vi "Autonomous Independent.vi"() -> ()   [LabVIEW 2015]
doc: "This VI is called when autonomous begins, and will automatically be terminated when autonomous ends. You can carry out timed or sensor driven robot movement independently without needing to return to the caller."
uses:
  <vilib>/Rock Robotics/WPI/Utilities/WPI_GetSetVariantRefNum.vi
  <vilib>/Rock Robotics/Network Tables/NT Read String.vi
  <vilib>/Rock Robotics/Network Tables/NT Write Numeric Array.vi
  <vilib>/Rock Robotics/Network Tables/NT Read Number.vi
  <vilib>/Rock Robotics/Network Tables/NT Write Number.vi
  <vilib>/addons/control/pid/pid.llb/PID (DBL).vi
  Robot Global Data.vi
  <vilib>/addons/control/pid/NI_PID_pid.lvlib
  navX Library v2/navX Library v2.lvlib
panel:
  out "E2 Rate 3":dbl
  out "E1 Rate 3":dbl
  out "Yaw 5":dbl(graph)
  out "Roll Display 3":dbl
  out "Pitch Display 3":dbl
  out "Yaw Display 3":dbl
  in  "Yaw 4":T1={"proportional gain (Kc)"=0.2, "integral time (Ti, min)"=0.0, "derivative time (Td, min)"=0.0} {"derivative time (Td, min)" format="%.3f"; "integral time (Ti, min)" format="%.3f"; "proportional gain (Kc)" format="%.3f"}
  out "Right Motor Speed  3":dbl(graph)
  out "Left Motor Speed 3":dbl(graph)
  in  "Speed Gains  3":T1={"proportional gain (Kc)"=0.65, "integral time (Ti, min)"=0.001, "derivative time (Td, min)"=0.001} {"derivative time (Td, min)" format="%.3f"; "integral time (Ti, min)" format="%.3f"; "proportional gain (Kc)" format="%.3f"}
  out "E2 Rate 2":dbl
  out "E1 Rate 2":dbl
  out "Yaw 3":dbl(graph)
  out "Roll Display 2":dbl
  out "Pitch Display 2":dbl
  out "Yaw Display 2":dbl
  in  "Yaw 2":T1={"proportional gain (Kc)"=0.2, "integral time (Ti, min)"=0.0, "derivative time (Td, min)"=0.0} {"derivative time (Td, min)" format="%.3f"; "integral time (Ti, min)" format="%.3f"; "proportional gain (Kc)" format="%.3f"}
  out "Right Motor Speed  2":dbl(graph)
  out "Left Motor Speed 2":dbl(graph)
  in  "Distance 2":dbl=120.0
  in  "Speed Gains  2":T1={"proportional gain (Kc)"=0.65, "integral time (Ti, min)"=0.001, "derivative time (Td, min)"=0.001} {"derivative time (Td, min)" format="%.3f"; "integral time (Ti, min)" format="%.3f"; "proportional gain (Kc)" format="%.3f"}
  out "Yaw Display":dbl
  out "Pitch Display":dbl
  out "Roll Display":dbl
  in  "Aiming Gains":T1={"proportional gain (Kc)"=1.0, "integral time (Ti, min)"=0.01, "derivative time (Td, min)"=0.0} {"derivative time (Td, min)" format="%.3f"; "integral time (Ti, min)" format="%.3f"; "proportional gain (Kc)" format="%.3f"}
  out "Yaw":dbl(graph)
  in  "Target Angle":dbl=30.0
  out "E1 Rate":dbl
  out "E2 Rate":dbl
  in  "Single Turn Gains":T1={"proportional gain (Kc)"=0.12, "integral time (Ti, min)"=0.0, "derivative time (Td, min)"=0.0} {"derivative time (Td, min)" format="%.3f"; "integral time (Ti, min)" format="%.3f"; "proportional gain (Kc)" format="%.3f"}
  in  "Yaw":T1={"proportional gain (Kc)"=0.2, "integral time (Ti, min)"=0.0, "derivative time (Td, min)"=0.0} {"derivative time (Td, min)" format="%.3f"; "integral time (Ti, min)" format="%.3f"; "proportional gain (Kc)" format="%.3f"}
  out "Right Motor Speed":dbl(graph)
  out "Left Motor Speed":dbl(graph)
  out "Right Motor":dbl(graph)
  out "Left Motor":dbl(graph)
  in  "Distance":dbl=120.0
  in  "Speed Gains":T1={"proportional gain (Kc)"=0.65, "integral time (Ti, min)"=0.001, "derivative time (Td, min)"=0.001} {"derivative time (Td, min)" format="%.3f"; "integral time (Ti, min)" format="%.3f"; "proportional gain (Kc)" format="%.3f"}
  out "E2 Dist":dbl
  out "E1 Dist":dbl
  # "Be sure to right-click and choose Data Operations>>Make Current Value default if you want to save the array values with the VI"
  # "Encoder Distance Traveled"
  # "Speed we are assigning the motors and Encoder Rate"
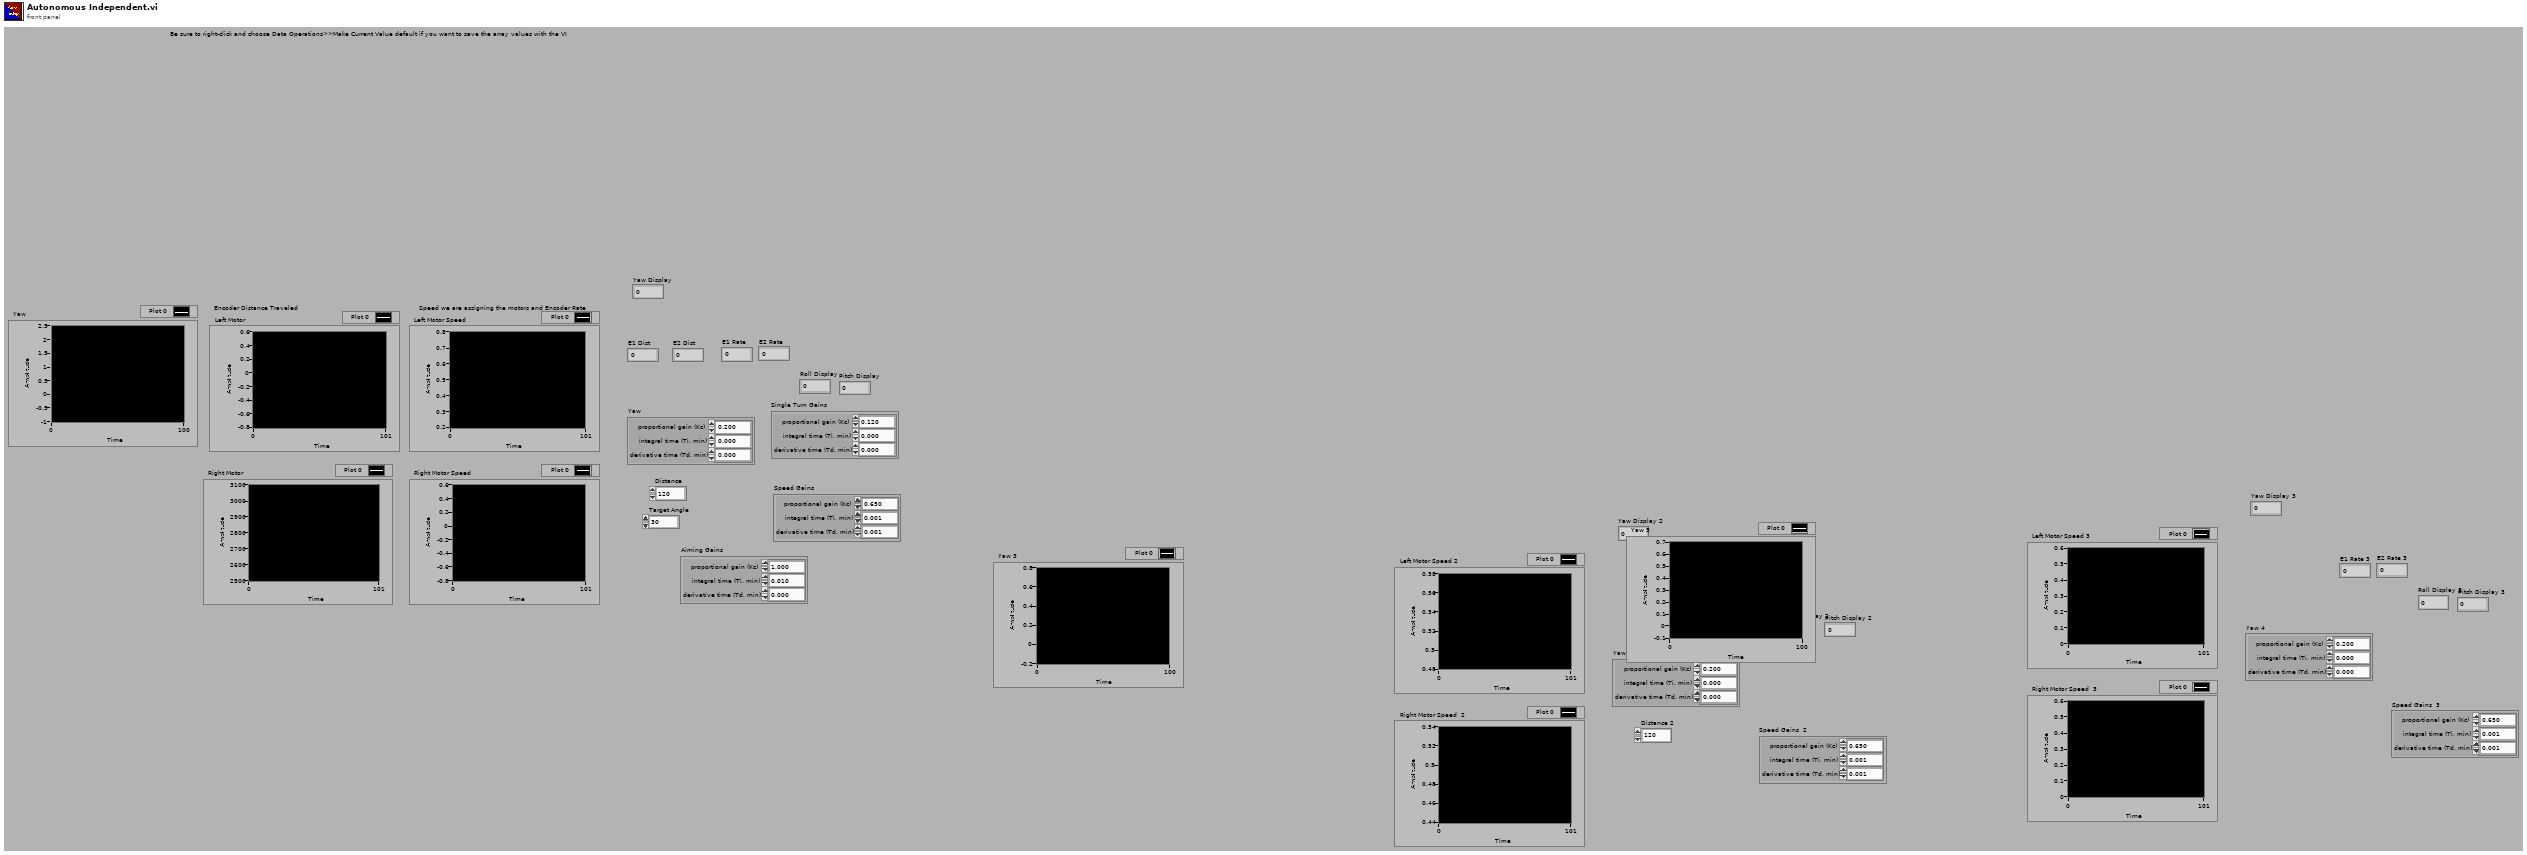
[diagram p1: front panel]
types:
  T1 = cluster{"proportional gain (Kc)":dbl, "integral time (Ti, min)":dbl, "derivative time (Td, min)":dbl}
  T2 = typedef "WPI_JoystickDevRef.ctl" = cluster{"Device":T3}
  T3 = typedef "WPI_JoystickDeviceEnum.ctl" = enum16{"USB 0", "USB 1", "USB 2", "USB 3", "USB 4", "USB 5"}
  T4 = typedef "navX Library v2.lvlib/Z900_navX_DeviceTypeDef.ctl" = cluster{"Interface":cluster{"Protocol":T5, "Update Rate (4Hz-60Hz)":u8, "navX Open TypeDef":variant}, "Notify Packet":refnum<notifier>, "Loop VI Refnum":refnum<vi>, "Ready to Close Occurrence Refnum":refnum<k4>}
  T5 = typedef "navX Library v2.lvlib/Z900_navX_ProtocolTypeDef.ctl" = enum16{"SERIAL", "I2C", "SPI"}
  T6 = typedef "WPI_EncoderDevRef.ctl" = cluster{"DevStatus":errorcluster, "EncoderIndex":T7, "CounterIndex":T8, "DistancePerCount":dbl, "Decoding Type":T9}
  T7 = typedef "FPGA_EncoderIdx.ctl" = enum8{"Enc 0", "Enc 1", "Enc 2", "Enc 3", "Enc 4", "Enc 5", "Enc 6", "Enc 7", "Invalid"}
  T8 = typedef "FPGA_CounterCtrSystemIndex.ctl" = enum8{"Ctr 0", "Ctr 1", "Ctr 2", "Ctr 3", "Ctr 4", "Ctr 5", "Ctr 6", "Ctr 7", "Invalid"}
  T9 = typedef "WPI_EncoderType.ctl" = enum16{"1x", "2x", "4x"}
  T10 = cluster{"Yaw":dbl, "Roll":dbl, "Pitch":dbl, "Heading":dbl, "Fused Heading":dbl}
  T11 = typedef "WPI_RobotDriveDevRef.ctl" = cluster{"DevStatus":errorcluster, "Motors[]":T12[], "Square Inputs":bool, "Max Output":dbl}
  T12 = typedef "WPI_MotorControlDeviceRef.ctl" = cluster{"DeviceStatus":errorcluster, "Type":T13, "PWM":cluster{"PWM Channel":T14, "DeadBand":T15}, "CAN":cluster{"Device Number":u8, "Control Mode":T16, "Semaphore":T17, "Max Vout":dbl, "TalonSRX Control Mode":T18}, "Invert":bool}
  T13 = typedef "WPI_MotorControlType.ctl" = enum16{"PWM", "CAN", "CANTalonSRX"}
  T14 = typedef "FPGA_DIOPWMChannel.ctl" = enum8{"PWM 0", "PWM 1", "PWM 2", "PWM 3", "PWM 4", "PWM 5", "PWM 6", "PWM 7", "PWM 8", "PWM 9", "PWM MXP 0", "PWM MXP 1", "PWM MXP 2", "PWM MXP 3", "PWM MXP 4", "PWM MXP 5", "PWM MXP 6", "PWM MXP 7", "PWM MXP 8", "PWM MXP 9", "Invalid"}
  T15 = typedef "WPI_PWMDeadband.ctl" = cluster{"Name":string, "maxPositivePwm":i32, "minPositivePwm":i32, "centerPwm":i32, "maxNegativePwm":i32, "minNegativePwm":i32, "angularRange":u16}
  T16 = typedef "WPI_CANJaguar_ControlMode.ctl" = enum8{"Percent VBus", "Current", "Speed", "Position", "Voltage"}
  T17 = typedef "Semaphore RefNum" = refnum<k1>
  T18 = typedef "WPI_CANTalonSRX_APIControlMode.ctl" = enum8{"Percent VBus", "Speed", "Position", "Slave", "Unchanged / Invalid", "Voltage Compensation", "Current", "Motion Profile"}
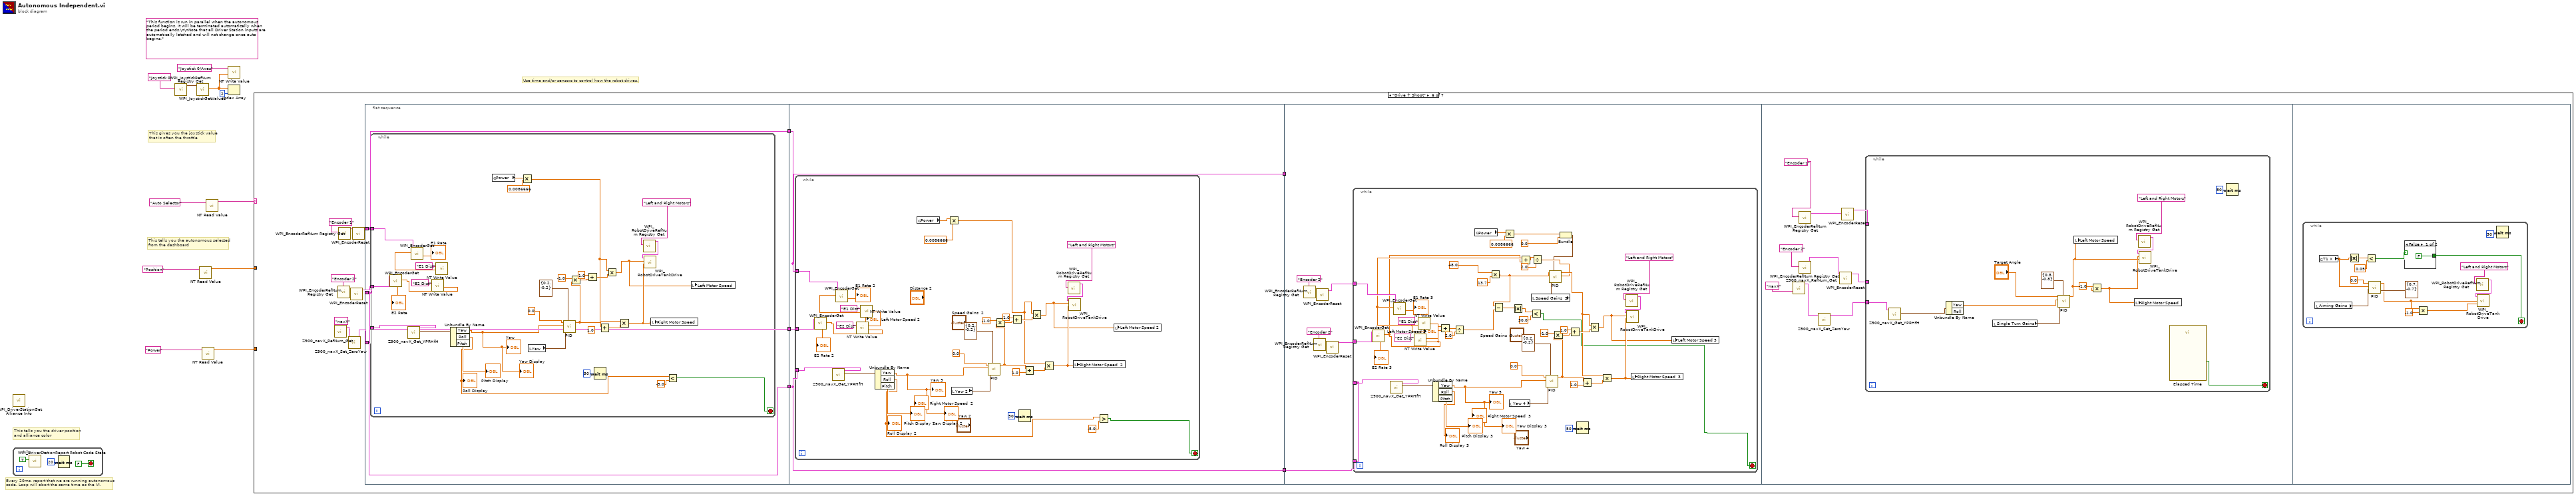
[diagram p0: block diagram]
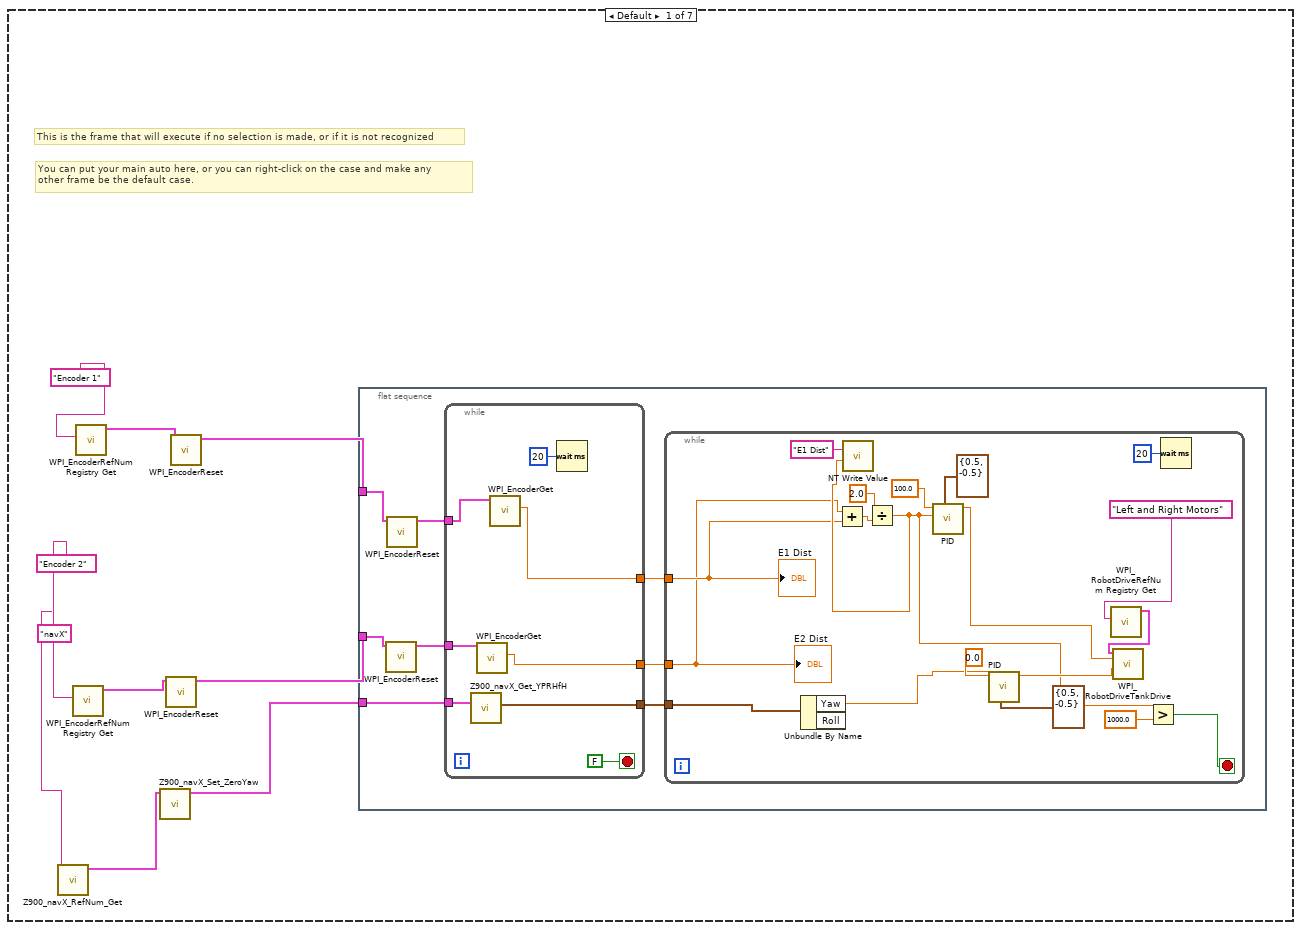
[diagram p2: hidden frame]
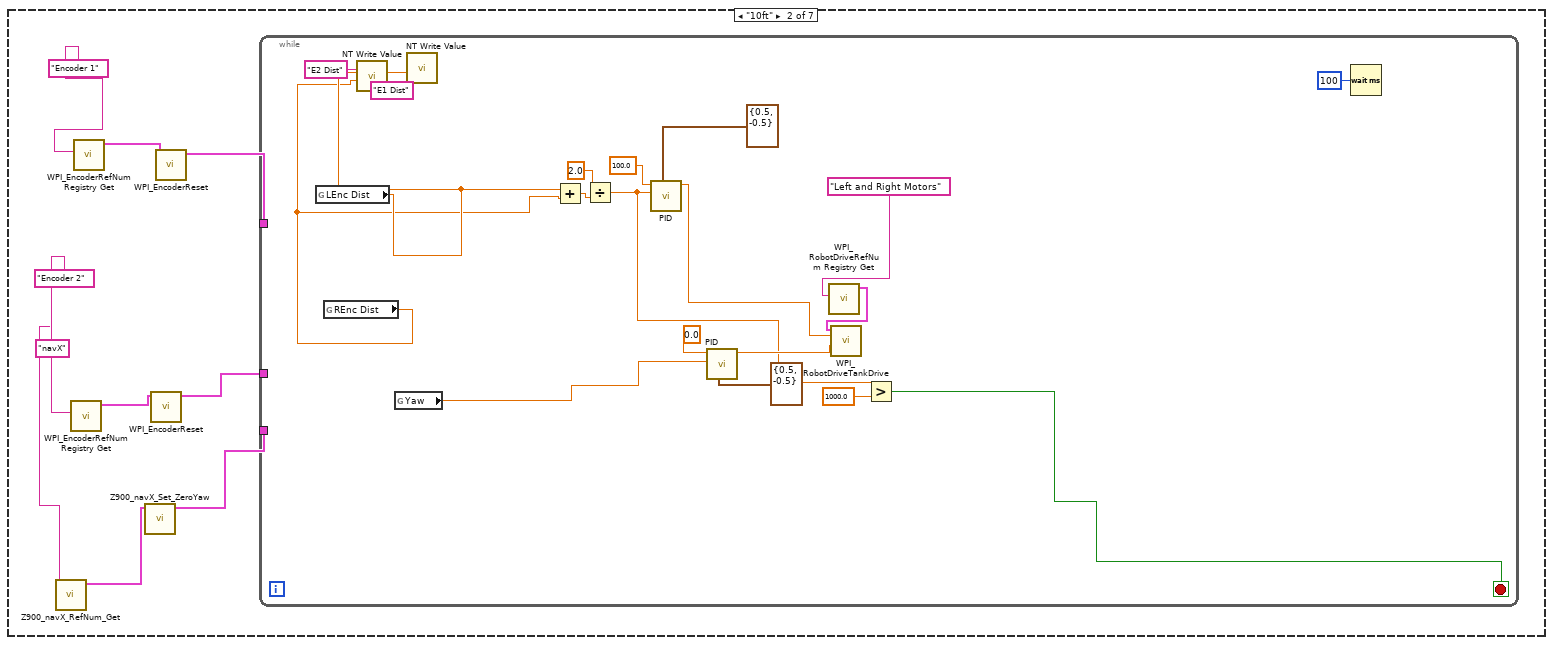
[diagram p3: hidden frame]
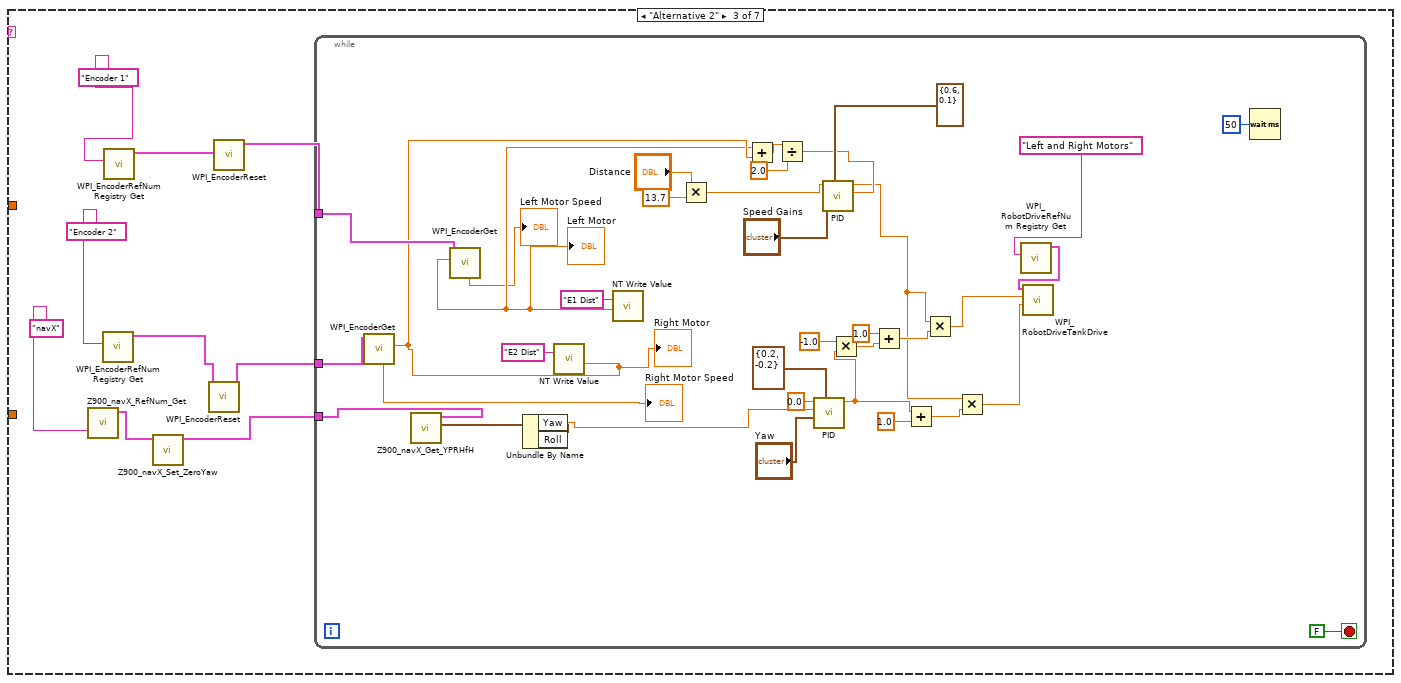
[diagram p4: hidden frame]
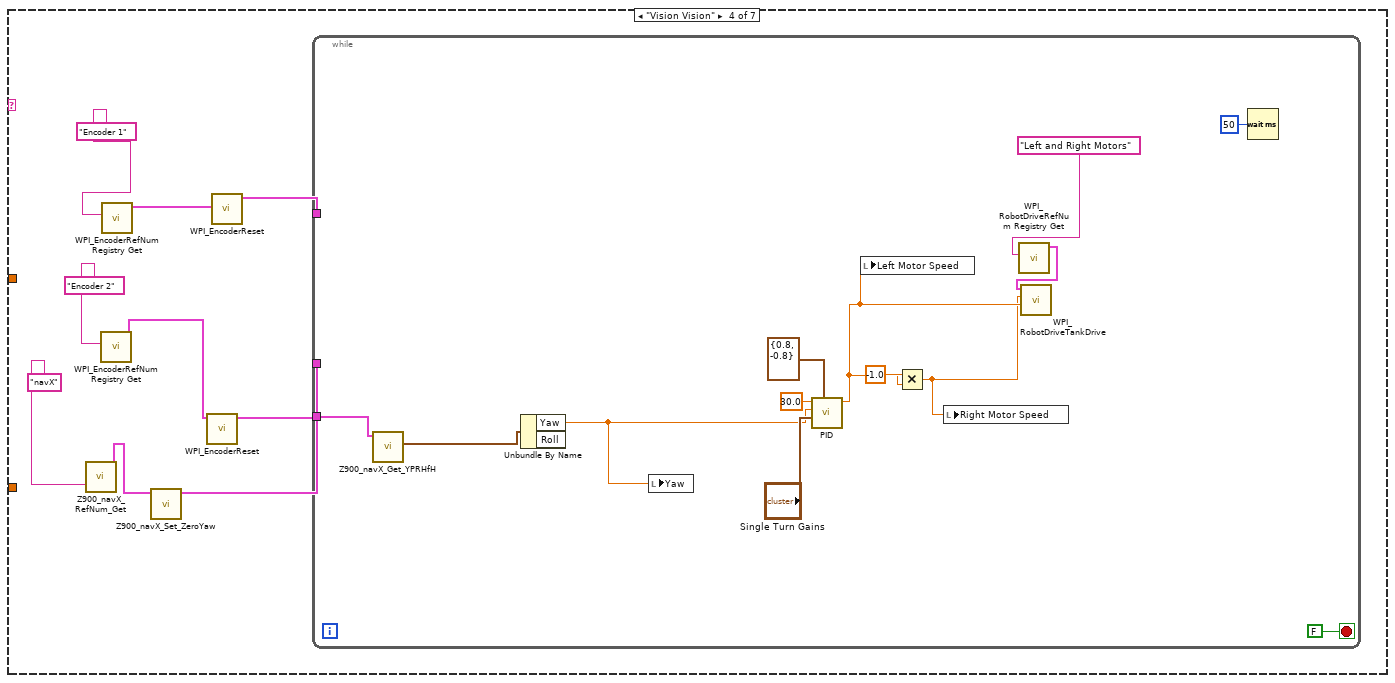
[diagram p5: hidden frame]
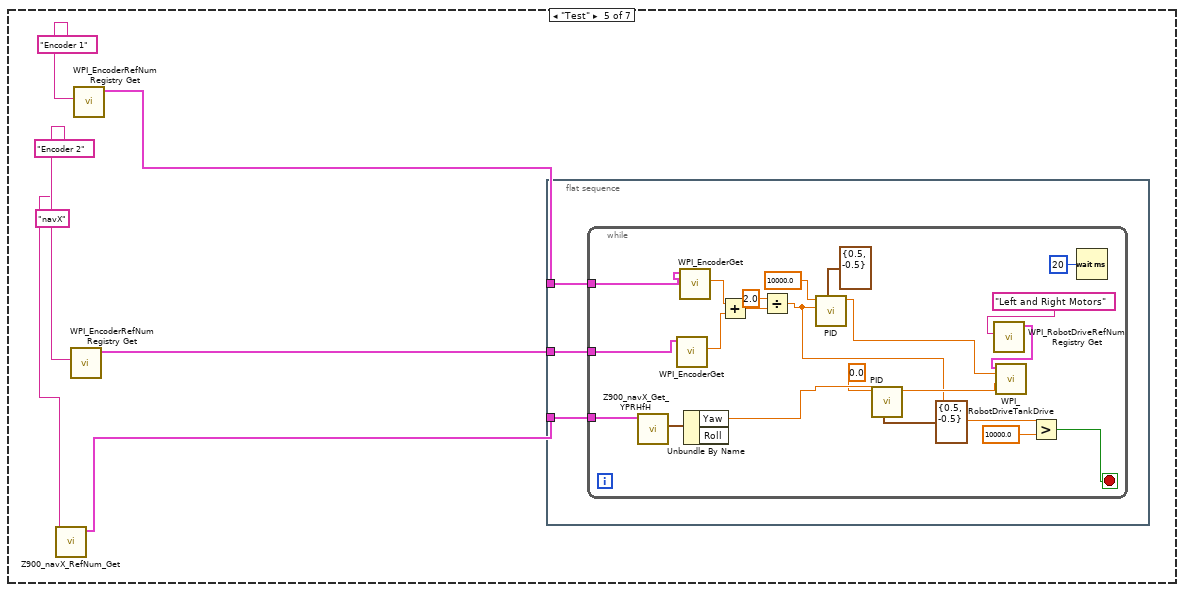
[diagram p6: hidden frame]
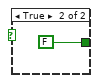
[diagram p7: hidden frame]
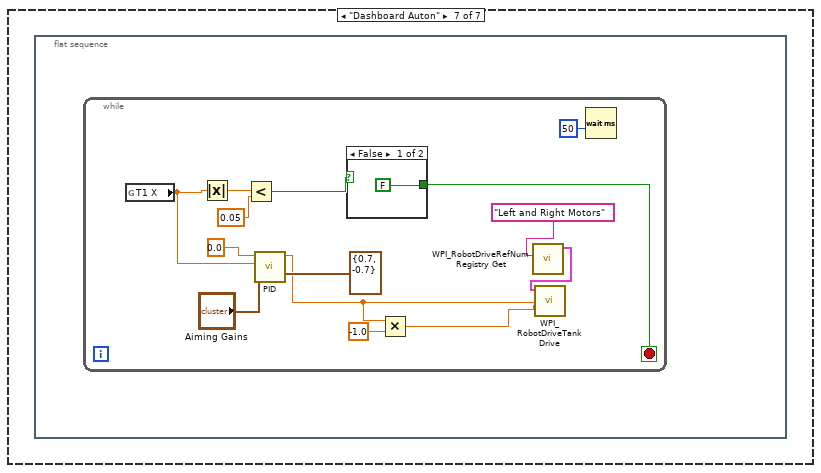
[diagram p8: hidden frame]
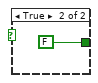
[diagram p9: hidden frame]
diagram:
  (unwired) "This function is run in parallel when the autonomous period begins. It will be terminated automatically when the period ends.\n\nNote that all Driver Station inputs are automatically latched and will not change once auto begins."
  # "This tells you the autonomous selected\nfrom the dashboard"
  # "Every 20ms, report that we are running autonomous\ncode. Loop will abort the same time as the VI."
  # "This gives you the joystick value\nthat is often the throttle"
  # "Use time and/or sensors to control how the robot drives."
  # "This tells you the driver position\nand alliance color"
  n1 = while {
    stop <- FALSE stop-if-true
    n2 = call <vilib>:"WPI_DriverStationReport Robot Code State.vi"("Autonomous"=TRUE) -> ()  [unwired: 10 in, 1 out]
    n3 = Wait (ms)(milliseconds to wait=u32 20) -> ()  [unwired: 1 out]
  }
  n4 = call <vilib>:"WPI_DriverStationGet Alliance Info.vi"() -> ()  [unwired: 12 out]
  n5 = call <vilib>:"WPI_JoystickRefNum Registry Get.vi"("refnum name"="Joystick 0") -> ("JoystickDevRef"=w10:T2)  [unwired: 1 in, 9 out]
  n6 = call <vilib>:"WPI_JoystickGetValues.vi"("JoystickDevRef"=w10) -> ("Axes"=w6:dbl[])  [unwired: 6 in, 4 out]
  n7 = call-poly <vilib>:"NT Read Value.vi"("Name"="Position") -> ("Numeric"=w2:dbl)  [unwired: 9 in, 1 out]
  n8 = call-poly <vilib>:"NT Read Value.vi"("Name"="Power") -> ("Numeric"=w1:dbl)  [unwired: 9 in, 1 out]
  n9 = call-poly <vilib>:"NT Read Value.vi"("Name"="Auto Selector") -> ("String"=w7:string)  [unwired: 9 in, 1 out]
  n10 = call-poly <vilib>:"NT Write Value.vi"("Numeric Array"=w6, "Name"="Joystick 0/Axes") -> ()  [unwired: 9 in, 1 out]
  n11 = Index Array(array=w6, index=2) -> ()  [unwired: 1 out]
  n12 = case shown="\"Drive + Shoot\"" w7 {
    tunnel: w2 -> [_ _ _ _ _ _ _]
    tunnel: w1 -> [_ _ _ _ _ _ _]
    frame Default {
      # "You can put your main auto here, or you can right-click on the case and make any\nother frame be the default case."
      # "This is the frame that will execute if no selection is made, or if it is not recognized"
      n13 = call "Z900_navX_RefNum_Get.vi"("refnum name"="navX") -> ("navX Device"=w17:T4)  [unwired: 9 in, 1 out]
      n14 = call <vilib>:"WPI_EncoderRefNum Registry Get.vi"("refnum name"="Encoder 2") -> ("EncoderDevRef"=w19:T6)  [unwired: 9 in, 1 out]
      n15 = call <vilib>:"WPI_EncoderRefNum Registry Get.vi"("refnum name"="Encoder 1") -> ("EncoderDevRef"=w21:T6)  [unwired: 9 in, 1 out]
      n16 = call "Z900_navX_Set_ZeroYaw.vi"("navX Device"=w17) -> ("navX Device"=w16:T4)  [unwired: 9 in, 1 out]
      n17 = call <vilib>:"WPI_EncoderReset.vi"("EncoderDevRef"=w19) -> ("EncoderDevRef"=w18:T6)  [unwired: 9 in, 1 out]
      n18 = call <vilib>:"WPI_EncoderReset.vi"("EncoderDevRef"=w21) -> ("EncoderDevRef"=w20:T6)  [unwired: 9 in, 1 out]
      n19 = flat-sequence {
        tunnel: w20 -> [w31]
        tunnel: w18 -> [w30]
        tunnel: w16 -> [w29]
        frame #0 {
          n20 = call <vilib>:"WPI_EncoderReset.vi"("EncoderDevRef"=w30) -> ("EncoderDevRef"=w28:T6)  [unwired: 9 in, 1 out]
          n21 = call <vilib>:"WPI_EncoderReset.vi"("EncoderDevRef"=w31) -> ("EncoderDevRef"=w27:T6)  [unwired: 9 in, 1 out]
          n22 = while {
            tunnel: w29 -> [w36]
            tunnel: w28 -> [w37]
            tunnel: w27 -> [w38]
            tunnel: [w35] -> w26
            tunnel: [w34] -> w25
            tunnel: [w33] -> w24
            stop <- FALSE stop-if-true
            n23 = call "Z900_navX_Get_YPRHfH.vi"("navX Device"=w36) -> ("YRPHfH"=w35:T10)  [unwired: 7 in, 3 out]
            n24 = call <vilib>:"WPI_EncoderGet.vi"("EncoderDevRef"=w37) -> ("Distance"=w34:dbl)  [unwired: 5 in, 5 out]
            n25 = call <vilib>:"WPI_EncoderGet.vi"("EncoderDevRef"=w38) -> ("Distance"=w33:dbl)  [unwired: 5 in, 5 out]
            n26 = Wait (ms)(milliseconds to wait=u32 20) -> ()  [unwired: 1 out]
          }
          n27 = while {
            tunnel: w26 -> [w43]
            tunnel: w25 -> [w41]
            tunnel: w24 -> [w42]
            stop <- w47 stop-if-true
            n28 = Unbundle By Name(w43) -> ("Yaw"=w44:dbl)  [unwired: 1 out]
            n29 = Add(x=w41, y=w42) -> (x+y=w58:dbl)
            n30 = Divide(x=2.0, y=w58) -> (x/y=w46:dbl)
            n31 = call-poly <vilib>:"NT Write Value.vi"("Numeric"=w46, "Name"="E1 Dist") -> ()  [unwired: 9 in, 1 out]
            n32 = call-poly <vilib>:"PID.vi"("output range"=cluster{"output high":dbl, "output low":dbl} {"output high"=0.5, "output low"=-0.5}, "process variable"=w46, "setpoint"=100.0) -> ("output"=w51:dbl)  [unwired: 7 in, 1 out]
            n33 = call-poly <vilib>:"PID.vi"("output range"=cluster{"output high":dbl, "output low":dbl} {"output high"=0.5, "output low"=-0.5}, "process variable"=w44, "setpoint"=0.0) -> ("output"=w50:dbl)  [unwired: 7 in, 1 out]
            n34 = call <vilib>:"WPI_RobotDriveRefNum Registry Get.vi"("refnum name"="Left and Right Motors") -> ("RobotDriveDevRef"=w53:T11)  [unwired: 9 in, 1 out]
            n35 = call <vilib>:"WPI_RobotDriveTankDrive.vi"("Right axis value"=w50, "Left axis value"=w51, "RobotDriveDevRef"=w53) -> ()  [unwired: 6 in, 3 out]
            n36 = Greater?(x=w46, y=1000.0) -> (0:w47:bool)
            n37 = Wait (ms)(milliseconds to wait=u32 20) -> ()  [unwired: 1 out]
            "E2 Dist" <- w41
            "E1 Dist" <- w42
          }
        }
      }
    }
    frame "10ft" {
      n38 = call "Z900_navX_RefNum_Get.vi"("refnum name"="navX") -> ("navX Device"=w61:T4)  [unwired: 9 in, 1 out]
      n39 = call <vilib>:"WPI_EncoderRefNum Registry Get.vi"("refnum name"="Encoder 2") -> ("EncoderDevRef"=w63:T6)  [unwired: 9 in, 1 out]
      n40 = call <vilib>:"WPI_EncoderRefNum Registry Get.vi"("refnum name"="Encoder 1") -> ("EncoderDevRef"=w65:T6)  [unwired: 9 in, 1 out]
      n41 = call "Z900_navX_Set_ZeroYaw.vi"("navX Device"=w61) -> ("navX Device"=w60:T4)  [unwired: 9 in, 1 out]
      n42 = call <vilib>:"WPI_EncoderReset.vi"("EncoderDevRef"=w63) -> ("EncoderDevRef"=w62:T6)  [unwired: 9 in, 1 out]
      n43 = call <vilib>:"WPI_EncoderReset.vi"("EncoderDevRef"=w65) -> ("EncoderDevRef"=w64:T6)  [unwired: 9 in, 1 out]
      n44 = while {
        tunnel: w64 -> [_]
        tunnel: w62 -> [_]
        tunnel: w60 -> [_]
        stop <- w68 stop-if-true
        n45 = global read "Robot Global Data.vi" "LEnc Dist"() -> (w71:dbl)
        n46 = global read "Robot Global Data.vi" "REnc Dist"() -> (w70:dbl)
        n47 = call-poly <vilib>:"NT Write Value.vi"("Numeric"=w70, "Name"="E2 Dist") -> ()  [unwired: 9 in, 1 out]
        n48 = global read "Robot Global Data.vi" "Yaw"() -> (w69:dbl)
        n49 = call-poly <vilib>:"NT Write Value.vi"("Numeric"=w71, "Name"="E1 Dist") -> ()  [unwired: 9 in, 1 out]
        n50 = Add(x=w71, y=w70) -> (x+y=w85:dbl)
        n51 = Divide(x=2.0, y=w85) -> (x/y=w75:dbl)
        n52 = call-poly <vilib>:"PID.vi"("output range"=cluster{"output high":dbl, "output low":dbl} {"output high"=0.5, "output low"=-0.5}, "process variable"=w75, "setpoint"=100.0) -> ("output"=w79:dbl)  [unwired: 7 in, 1 out]
        n53 = call-poly <vilib>:"PID.vi"("output range"=cluster{"output high":dbl, "output low":dbl} {"output high"=0.5, "output low"=-0.5}, "process variable"=w69, "setpoint"=0.0) -> ("output"=w78:dbl)  [unwired: 7 in, 1 out]
        n54 = call <vilib>:"WPI_RobotDriveRefNum Registry Get.vi"("refnum name"="Left and Right Motors") -> ("RobotDriveDevRef"=w81:T11)  [unwired: 9 in, 1 out]
        n55 = call <vilib>:"WPI_RobotDriveTankDrive.vi"("Right axis value"=w78, "Left axis value"=w79, "RobotDriveDevRef"=w81) -> ()  [unwired: 6 in, 3 out]
        n56 = Greater?(x=w75, y=1000.0) -> (0:w68:bool)
        n57 = Wait (ms)(milliseconds to wait=u32 100) -> ()  [unwired: 1 out]
      }
    }
    frame "Alternative 2" {
      n58 = call "Z900_navX_RefNum_Get.vi"("refnum name"="navX") -> ("navX Device"=w88:T4)  [unwired: 9 in, 1 out]
      n59 = call <vilib>:"WPI_EncoderRefNum Registry Get.vi"("refnum name"="Encoder 2") -> ("EncoderDevRef"=w90:T6)  [unwired: 9 in, 1 out]
      n60 = call <vilib>:"WPI_EncoderRefNum Registry Get.vi"("refnum name"="Encoder 1") -> ("EncoderDevRef"=w92:T6)  [unwired: 9 in, 1 out]
      n61 = call "Z900_navX_Set_ZeroYaw.vi"("navX Device"=w88) -> ("navX Device"=w87:T4)  [unwired: 9 in, 1 out]
      n62 = call <vilib>:"WPI_EncoderReset.vi"("EncoderDevRef"=w90) -> ("EncoderDevRef"=w89:T6)  [unwired: 9 in, 1 out]
      n63 = call <vilib>:"WPI_EncoderReset.vi"("EncoderDevRef"=w92) -> ("EncoderDevRef"=w91:T6)  [unwired: 9 in, 1 out]
      n64 = while {
        tunnel: w91 -> [w124]
        tunnel: w89 -> [w123]
        tunnel: w87 -> [w122]
        stop <- FALSE stop-if-true
        n65 = call <vilib>:"WPI_EncoderGet.vi"("EncoderDevRef"=w123) -> ("Distance"=w113:dbl, "Rate"=→"Right Motor Speed":dbl)  [unwired: 5 in, 4 out]
        "Right Motor" <- w113
        n66 = call "Z900_navX_Get_YPRHfH.vi"("navX Device"=w122) -> ("YRPHfH"=w125:T10)  [unwired: 7 in, 3 out]
        n67 = call <vilib>:"WPI_EncoderGet.vi"("EncoderDevRef"=w124) -> ("Distance"=w112:dbl, "Rate"=→"Left Motor Speed":dbl)  [unwired: 5 in, 4 out]
        "Left Motor" <- w112
        n68 = Unbundle By Name(w125) -> ("Yaw"=w98:dbl)  [unwired: 1 out]
        n69 = call-poly <vilib>:"NT Write Value.vi"("Numeric"=w113, "Name"="E2 Dist") -> ()  [unwired: 9 in, 1 out]
        n70 = call-poly <vilib>:"NT Write Value.vi"("Numeric"=w112, "Name"="E1 Dist") -> ()  [unwired: 9 in, 1 out]
        n71 = Multiply(x="Distance", y=13.7) -> (x*y=w114:dbl)
        n72 = Add(x=w112, y=w113) -> (x+y=w119:dbl)
        n73 = Divide(x=w119, y=2.0) -> (x/y=w117:dbl)
        n74 = call-poly <vilib>:"PID.vi"("output range"=cluster{"output high":dbl, "output low":dbl} {"output high"=0.2, "output low"=-0.2}, "PID gains"="Yaw", "process variable"=w98, "setpoint"=0.0) -> ("output"=w102:dbl)  [unwired: 6 in, 1 out]
        n75 = call-poly <vilib>:"PID.vi"("output range"=cluster{"output high":dbl, "output low":dbl} {"output high"=0.6, "output low"=0.1}, "PID gains"="Speed Gains", "process variable"=w117, "setpoint"=w114) -> ("output"=w99:dbl)  [unwired: 6 in, 1 out]
        n76 = Multiply(x=-1.0, y=w102) -> (x*y=w103:dbl)
        n77 = Add(x=1.0, y=w103) -> (x+y=w104:dbl)
        n78 = Add(x=w102, y=1.0) -> (x+y=w105:dbl)
        n79 = Multiply(x=w99, y=w104) -> (x*y=w96:dbl)
        n80 = Multiply(x=w99, y=w105) -> (x*y=w97:dbl)
        n81 = call <vilib>:"WPI_RobotDriveRefNum Registry Get.vi"("refnum name"="Left and Right Motors") -> ("RobotDriveDevRef"=w127:T11)  [unwired: 9 in, 1 out]
        n82 = call <vilib>:"WPI_RobotDriveTankDrive.vi"("Right axis value"=w97, "Left axis value"=w96, "RobotDriveDevRef"=w127) -> ()  [unwired: 6 in, 3 out]
        n83 = Wait (ms)(milliseconds to wait=u32 50) -> ()  [unwired: 1 out]
      }
    }
    frame "Vision Vision" {
      n84 = call "Z900_navX_RefNum_Get.vi"("refnum name"="navX") -> ("navX Device"=w133:T4)  [unwired: 9 in, 1 out]
      n85 = call <vilib>:"WPI_EncoderRefNum Registry Get.vi"("refnum name"="Encoder 2") -> ("EncoderDevRef"=w135:T6)  [unwired: 9 in, 1 out]
      n86 = call <vilib>:"WPI_EncoderRefNum Registry Get.vi"("refnum name"="Encoder 1") -> ("EncoderDevRef"=w137:T6)  [unwired: 9 in, 1 out]
      n87 = call "Z900_navX_Set_ZeroYaw.vi"("navX Device"=w133) -> ("navX Device"=w132:T4)  [unwired: 9 in, 1 out]
      n88 = call <vilib>:"WPI_EncoderReset.vi"("EncoderDevRef"=w135) -> ("EncoderDevRef"=w134:T6)  [unwired: 9 in, 1 out]
      n89 = call <vilib>:"WPI_EncoderReset.vi"("EncoderDevRef"=w137) -> ("EncoderDevRef"=w136:T6)  [unwired: 9 in, 1 out]
      n90 = while {
        tunnel: w136 -> [_]
        tunnel: w134 -> [_]
        tunnel: w132 -> [w147]
        stop <- FALSE stop-if-true
        n91 = call "Z900_navX_Get_YPRHfH.vi"("navX Device"=w147) -> ("YRPHfH"=w146:T10)  [unwired: 7 in, 3 out]
        n92 = Unbundle By Name(w146) -> ("Yaw"=w141:dbl)  [unwired: 1 out]
        n93 = local write "Yaw"(w141) -> ()
        n94 = call-poly <vilib>:"PID.vi"("output range"=cluster{"output high":dbl, "output low":dbl} {"output high"=0.8, "output low"=-0.8}, "PID gains"="Single Turn Gains", "process variable"=w141, "setpoint"=30.0) -> ("output"=w143:dbl)  [unwired: 6 in, 1 out]
        n95 = local write "Left Motor Speed"(w143) -> ()
        n96 = Multiply(x=-1.0, y=w143) -> (x*y=w142:dbl)
        n97 = local write "Right Motor Speed"(w142) -> ()
        n98 = call <vilib>:"WPI_RobotDriveRefNum Registry Get.vi"("refnum name"="Left and Right Motors") -> ("RobotDriveDevRef"=w152:T11)  [unwired: 9 in, 1 out]
        n99 = call <vilib>:"WPI_RobotDriveTankDrive.vi"("Right axis value"=w143, "Left axis value"=w142, "RobotDriveDevRef"=w152) -> ()  [unwired: 6 in, 3 out]
        n100 = Wait (ms)(milliseconds to wait=u32 50) -> ()  [unwired: 1 out]
      }
    }
    frame "Test" {
      n101 = call "Z900_navX_RefNum_Get.vi"("refnum name"="navX") -> ("navX Device"=w154:T4)  [unwired: 9 in, 1 out]
      n102 = call <vilib>:"WPI_EncoderRefNum Registry Get.vi"("refnum name"="Encoder 2") -> ("EncoderDevRef"=w155:T6)  [unwired: 9 in, 1 out]
      n103 = call <vilib>:"WPI_EncoderRefNum Registry Get.vi"("refnum name"="Encoder 1") -> ("EncoderDevRef"=w156:T6)  [unwired: 9 in, 1 out]
      n104 = flat-sequence {
        tunnel: w156 -> [w162]
        tunnel: w155 -> [w161]
        tunnel: w154 -> [w160]
        frame #0 {
          n105 = while {
            tunnel: w162 -> [w182]
            tunnel: w161 -> [w181]
            tunnel: w160 -> [w172]
            stop <- w163 stop-if-true
            n106 = call "Z900_navX_Get_YPRHfH.vi"("navX Device"=w172) -> ("YRPHfH"=w183:T10)  [unwired: 7 in, 3 out]
            n107 = call <vilib>:"WPI_EncoderGet.vi"("EncoderDevRef"=w181) -> ("Distance"=w178:dbl)  [unwired: 5 in, 5 out]
            n108 = call <vilib>:"WPI_EncoderGet.vi"("EncoderDevRef"=w182) -> ("Distance"=w179:dbl)  [unwired: 5 in, 5 out]
            n109 = Unbundle By Name(w183) -> ("Yaw"=w174:dbl)  [unwired: 1 out]
            n110 = Add(x=w179, y=w178) -> (x+y=w177:dbl)
            n111 = Divide(x=2.0, y=w177) -> (x/y=w165:dbl)
            n112 = call-poly <vilib>:"PID.vi"("output range"=cluster{"output high":dbl, "output low":dbl} {"output high"=0.5, "output low"=-0.5}, "process variable"=w165, "setpoint"=10000.0) -> ("output"=w168:dbl)  [unwired: 7 in, 1 out]
            n113 = call-poly <vilib>:"PID.vi"("output range"=cluster{"output high":dbl, "output low":dbl} {"output high"=0.5, "output low"=-0.5}, "process variable"=w174, "setpoint"=0.0) -> ("output"=w167:dbl)  [unwired: 7 in, 1 out]
            n114 = call <vilib>:"WPI_RobotDriveRefNum Registry Get.vi"("refnum name"="Left and Right Motors") -> ("RobotDriveDevRef"=w170:T11)  [unwired: 9 in, 1 out]
            n115 = call <vilib>:"WPI_RobotDriveTankDrive.vi"("Right axis value"=w167, "Left axis value"=w168, "RobotDriveDevRef"=w170) -> ()  [unwired: 6 in, 3 out]
            n116 = Greater?(x=w165, y=10000.0) -> (0:w163:bool)
            n117 = Wait (ms)(milliseconds to wait=u32 20) -> ()  [unwired: 1 out]
          }
        }
      }
    }
    frame "Drive + Shoot" {
      n118 = call "Z900_navX_RefNum_Get.vi"("refnum name"="navX") -> ("navX Device"=w196:T4)  [unwired: 9 in, 1 out]
      n119 = call <vilib>:"WPI_EncoderRefNum Registry Get.vi"("refnum name"="Encoder 2") -> ("EncoderDevRef"=w194:T6)  [unwired: 9 in, 1 out]
      n120 = call <vilib>:"WPI_EncoderRefNum Registry Get.vi"("refnum name"="Encoder 1") -> ("EncoderDevRef"=w192:T6)  [unwired: 9 in, 1 out]
      n121 = call "Z900_navX_Set_ZeroYaw.vi"("navX Device"=w196) -> ("navX Device"=w197:T4)  [unwired: 9 in, 1 out]
      n122 = call <vilib>:"WPI_EncoderReset.vi"("EncoderDevRef"=w194) -> ("EncoderDevRef"=w195:T6)  [unwired: 9 in, 1 out]
      n123 = call <vilib>:"WPI_EncoderReset.vi"("EncoderDevRef"=w192) -> ("EncoderDevRef"=w193:T6)  [unwired: 9 in, 1 out]
      n124 = flat-sequence {
        tunnel: w197 -> [w200]
        tunnel: w195 -> [w199]
        tunnel: w193 -> [w198]
        tunnel: [w200] -> w188
        tunnel: [w199] -> w187
        tunnel: [w198] -> w186
        tunnel: [w236] -> w185
        tunnel: [w235] -> w184
        tunnel: w186 -> [w235]
        tunnel: w187 -> [w234]
        tunnel: w188 -> [w236]
        tunnel: w185 -> [w276]
        tunnel: w184 -> [_]
        frame #0 {
          n125 = while {
            tunnel: w198 -> [w227]
            tunnel: w199 -> [w226]
            tunnel: w200 -> [w225]
            stop <- w202 stop-if-true
            n126 = call <vilib>:"WPI_EncoderGet.vi"("EncoderDevRef"=w226) -> ("Distance"=w209:dbl, "Rate"=→"E2 Rate":dbl)  [unwired: 5 in, 4 out]
            n127 = call "Z900_navX_Get_YPRHfH.vi"("navX Device"=w225) -> ("YRPHfH"=w228:T10)  [unwired: 7 in, 3 out]
            n128 = call <vilib>:"WPI_EncoderGet.vi"("EncoderDevRef"=w227) -> ("Distance"=w210:dbl, "Rate"=→"E1 Rate":dbl)  [unwired: 5 in, 4 out]
            n129 = call-poly <vilib>:"NT Write Value.vi"("Numeric"=w209, "Name"="E2 Dist") -> ()  [unwired: 9 in, 1 out]
            n130 = call-poly <vilib>:"NT Write Value.vi"("Numeric"=w210, "Name"="E1 Dist") -> ()  [unwired: 9 in, 1 out]
            n131 = Unbundle By Name(w228) -> ("Yaw"=w205:dbl, "Roll"=w204:dbl, "Pitch"=→"Pitch Display":dbl)
            "Yaw" <- w205
            "Roll Display" <- w204
            "Yaw Display" <- w205
            n132 = global read "Robot Global Data.vi" "Power"() -> (w207:dbl)
            n133 = Multiply(x=w207, y=0.0086666) -> (x*y=w201:dbl)
            n134 = local read "Yaw"() -> (w215:T1)
            n135 = call-poly <vilib>:"PID.vi"("output range"=cluster{"output high":dbl, "output low":dbl} {"output high"=0.2, "output low"=-0.2}, "PID gains"=w215, "process variable"=w205, "setpoint"=0.0) -> ("output"=w219:dbl)  [unwired: 6 in, 1 out]
            n136 = Multiply(x=-1.0, y=w219) -> (x*y=w220:dbl)
            n137 = Add(x=1.0, y=w220) -> (x+y=w221:dbl)
            n138 = Wait (ms)(milliseconds to wait=u32 50) -> ()  [unwired: 1 out]
            n139 = Add(x=w219, y=1.0) -> (x+y=w222:dbl)
            n140 = Multiply(x=w201, y=w221) -> (x*y=w212:dbl)
            n141 = Multiply(x=w201, y=w222) -> (x*y=w214:dbl)
            n142 = call <vilib>:"WPI_RobotDriveRefNum Registry Get.vi"("refnum name"="Left and Right Motors") -> ("RobotDriveDevRef"=w230:T11)  [unwired: 9 in, 1 out]
            n143 = call <vilib>:"WPI_RobotDriveTankDrive.vi"("Right axis value"=w214, "Left axis value"=w212, "RobotDriveDevRef"=w230) -> ()  [unwired: 6 in, 3 out]
            n144 = local write "Right Motor Speed"(w214) -> ()
            n145 = Less?(x=w204, y=-5.0) -> (x < y?=w202:bool)
            n146 = local write "Left Motor Speed"(w212) -> ()
          }
        }
        frame #1 {
          n147 = while {
            tunnel: w235 -> [w263]
            tunnel: w234 -> [w262]
            tunnel: w236 -> [w261]
            stop <- w242 stop-if-true
            n148 = call <vilib>:"WPI_EncoderGet.vi"("EncoderDevRef"=w262) -> ("Distance"=w245:dbl, "Rate"=→"E2 Rate 2":dbl)  [unwired: 5 in, 4 out]
            n149 = call "Z900_navX_Get_YPRHfH.vi"("navX Device"=w261) -> ("YRPHfH"=w264:T10)  [unwired: 7 in, 3 out]
            n150 = call <vilib>:"WPI_EncoderGet.vi"("EncoderDevRef"=w263) -> ("Distance"=w246:dbl, "Rate"=→"E1 Rate 2":dbl)  [unwired: 5 in, 4 out]
            n151 = call-poly <vilib>:"NT Write Value.vi"("Numeric"=w245, "Name"="E2 Dist") -> ()  [unwired: 9 in, 1 out]
            n152 = call-poly <vilib>:"NT Write Value.vi"("Numeric"=w246, "Name"="E1 Dist") -> ()  [unwired: 9 in, 1 out]
            n153 = Unbundle By Name(w264) -> ("Yaw"=w243:dbl, "Roll"=w241:dbl, "Pitch"=→"Pitch Display 2":dbl)
            "Yaw 3" <- w243
            "Roll Display 2" <- w241
            "Yaw Display 2" <- w243
            n154 = global read "Robot Global Data.vi" "Power"() -> (w238:dbl)
            n155 = Multiply(x=w238, y=0.0086666) -> (x*y=w237:dbl)
            n156 = local read "Yaw 2"() -> (w251:T1)
            n157 = call-poly <vilib>:"PID.vi"("output range"=cluster{"output high":dbl, "output low":dbl} {"output high"=0.2, "output low"=-0.2}, "PID gains"=w251, "process variable"=w243, "setpoint"=0.0) -> ("output"=w255:dbl)  [unwired: 6 in, 1 out]
            n158 = Multiply(x=-1.0, y=w255) -> (x*y=w256:dbl)
            n159 = Add(x=1.0, y=w256) -> (x+y=w257:dbl)
            n160 = Wait (ms)(milliseconds to wait=u32 50) -> ()  [unwired: 1 out]
            n161 = Add(x=w255, y=1.0) -> (x+y=w258:dbl)
            n162 = Multiply(x=w237, y=w257) -> (x*y=w248:dbl)
            n163 = Multiply(x=w237, y=w258) -> (x*y=w250:dbl)
            n164 = call <vilib>:"WPI_RobotDriveRefNum Registry Get.vi"("refnum name"="Left and Right Motors") -> ("RobotDriveDevRef"=w266:T11)  [unwired: 9 in, 1 out]
            n165 = call <vilib>:"WPI_RobotDriveTankDrive.vi"("Right axis value"=w250, "Left axis value"=w248, "RobotDriveDevRef"=w266) -> ()  [unwired: 6 in, 3 out]
            n166 = local write "Right Motor Speed  2"(w250) -> ()
            n167 = Greater?(x=w241, y=-5.0) -> (0:w242:bool)
            n168 = local write "Left Motor Speed 2"(w248) -> ()
          }
        }
        frame #2 {
          n169 = call <vilib>:"WPI_EncoderRefNum Registry Get.vi"("refnum name"="Encoder 2") -> ("EncoderDevRef"=w272:T6)  [unwired: 9 in, 1 out]
          n170 = call <vilib>:"WPI_EncoderRefNum Registry Get.vi"("refnum name"="Encoder 2") -> ("EncoderDevRef"=w275:T6)  [unwired: 9 in, 1 out]
          n171 = call <vilib>:"WPI_EncoderReset.vi"("EncoderDevRef"=w272) -> ("EncoderDevRef"=w270:T6)  [unwired: 9 in, 1 out]
          n172 = call <vilib>:"WPI_EncoderReset.vi"("EncoderDevRef"=w275) -> ("EncoderDevRef"=w273:T6)  [unwired: 9 in, 1 out]
          n173 = while {
            tunnel: w270 -> [w318]
            tunnel: [w289] -> _
            tunnel: w276 -> [w289]
            tunnel: w273 -> [w288]
            stop <- w278 stop-if-true
            n174 = call <vilib>:"WPI_EncoderGet.vi"("EncoderDevRef"=w288) -> ("Distance"=w284:dbl, "Rate"=→"E2 Rate 3":dbl)  [unwired: 5 in, 4 out]
            n175 = call "Z900_navX_Get_YPRHfH.vi"("navX Device"=w289) -> ("YRPHfH"=w319:T10)  [unwired: 7 in, 3 out]
            n176 = call <vilib>:"WPI_EncoderGet.vi"("EncoderDevRef"=w318) -> ("Distance"=w285:dbl, "Rate"=→"E1 Rate 3":dbl)  [unwired: 5 in, 4 out]
            n177 = call-poly <vilib>:"NT Write Value.vi"("Numeric"=w284, "Name"="E2 Dist") -> ()  [unwired: 9 in, 1 out]
            n178 = call-poly <vilib>:"NT Write Value.vi"("Numeric"=w285, "Name"="E1 Dist") -> ()  [unwired: 9 in, 1 out]
            n179 = Unbundle By Name(w319) -> ("Yaw"=w292:dbl, "Roll"=→"Roll Display 3":dbl, "Pitch"=→"Pitch Display 3":dbl)
            "Yaw 5" <- w292
            "Yaw Display 3" <- w292
            n180 = Add(x=w285, y=w284) -> (x+y=w287:dbl)
            n181 = Divide(x=w287, y=2.0) -> (x/y=w283:dbl)
            n182 = global read "Robot Global Data.vi" "Power"() -> (w295:dbl)
            n183 = Multiply(x=48.0, y=13.7) -> (x*y=w282:dbl)
            n184 = Subtract(x=w282, y=w283) -> (x-y=w281:dbl)
            n185 = Multiply(x=w295, y=0.0086666) -> (x*y=w294:dbl)
            n186 = local read "Yaw 4"() -> (w305:T1)
            n187 = Absolute Value(x=w281) -> (abs(x)=w280:dbl)
            n188 = Add(x=w285, y=w284) -> (x+y=w317:dbl)
            n189 = Less?(x=w280, y=30.0) -> (x < y?=w278:bool)
            n190 = Divide(x=w317, y=2.0) -> (x/y=w299:dbl)
            n191 = local read "Speed Gains  3"() -> (w301:T1)
            n192 = call-poly <vilib>:"PID.vi"("output range"=cluster{"output high":dbl, "output low":dbl} {"output high"=0.2, "output low"=-0.2}, "PID gains"=w305, "process variable"=w292, "setpoint"=0.0) -> ("output"=w310:dbl)  [unwired: 6 in, 1 out]
            n193 = Multiply(x=-1.0, y=w310) -> (x*y=w311:dbl)
            n194 = Bundle(w294, 0.0) -> (w297:cluster{dbl, dbl})  [unwired: 1 in]
            n195 = call-poly <vilib>:"PID.vi"("output range"=w297, "PID gains"=w301, "process variable"=w299, "setpoint"=w282) -> ("output"=w307:dbl)  [unwired: 6 in, 1 out]
            n196 = Add(x=1.0, y=w311) -> (x+y=w312:dbl)
            n197 = Wait (ms)(milliseconds to wait=u32 50) -> ()  [unwired: 1 out]
            n198 = Add(x=w310, y=1.0) -> (x+y=w313:dbl)
            n199 = Multiply(x=w307, y=w312) -> (x*y=w302:dbl)
            n200 = Multiply(x=w307, y=w313) -> (x*y=w304:dbl)
            n201 = call <vilib>:"WPI_RobotDriveRefNum Registry Get.vi"("refnum name"="Left and Right Motors") -> ("RobotDriveDevRef"=w321:T11)  [unwired: 9 in, 1 out]
            n202 = call <vilib>:"WPI_RobotDriveTankDrive.vi"("Right axis value"=w304, "Left axis value"=w302, "RobotDriveDevRef"=w321) -> ()  [unwired: 6 in, 3 out]
            n203 = local write "Right Motor Speed  3"(w304) -> ()
            n204 = local write "Left Motor Speed 3"(w302) -> ()
          }
        }
        frame #3 {
          n205 = call "Z900_navX_RefNum_Get.vi"("refnum name"="navX") -> ("navX Device"=w326:T4)  [unwired: 9 in, 1 out]
          n206 = call <vilib>:"WPI_EncoderRefNum Registry Get.vi"("refnum name"="Encoder 2") -> ("EncoderDevRef"=w328:T6)  [unwired: 9 in, 1 out]
          n207 = call <vilib>:"WPI_EncoderRefNum Registry Get.vi"("refnum name"="Encoder 1") -> ("EncoderDevRef"=w330:T6)  [unwired: 9 in, 1 out]
          n208 = call "Z900_navX_Set_ZeroYaw.vi"("navX Device"=w326) -> ("navX Device"=w325:T4)  [unwired: 9 in, 1 out]
          n209 = call <vilib>:"WPI_EncoderReset.vi"("EncoderDevRef"=w328) -> ("EncoderDevRef"=w327:T6)  [unwired: 9 in, 1 out]
          n210 = call <vilib>:"WPI_EncoderReset.vi"("EncoderDevRef"=w330) -> ("EncoderDevRef"=w329:T6)  [unwired: 9 in, 1 out]
          n211 = while {
            tunnel: w329 -> [_]
            tunnel: w327 -> [_]
            tunnel: w325 -> [w342]
            stop <- w334 stop-if-true
            n212 = call "Z900_navX_Get_YPRHfH.vi"("navX Device"=w342) -> ("YRPHfH"=w341:T10)  [unwired: 7 in, 3 out]
            n213 = Unbundle By Name(w341) -> ("Yaw"=w339:dbl)  [unwired: 1 out]
            n214 = local read "Single Turn Gains"() -> (w337:T1)
            n215 = call-poly <vilib>:"PID.vi"("output range"=cluster{"output high":dbl, "output low":dbl} {"output high"=0.8, "output low"=-0.8}, "PID gains"=w337, "process variable"=w339, "setpoint"="Target Angle") -> ("output"=w336:dbl)  [unwired: 6 in, 1 out]
            n216 = local write "Left Motor Speed"(w336) -> ()
            n217 = Multiply(x=-1.0, y=w336) -> (x*y=w335:dbl)
            n218 = local write "Right Motor Speed"(w335) -> ()
            n219 = call <vilib>:"WPI_RobotDriveRefNum Registry Get.vi"("refnum name"="Left and Right Motors") -> ("RobotDriveDevRef"=w345:T11)  [unwired: 9 in, 1 out]
            n220 = call <vilib>:"WPI_RobotDriveTankDrive.vi"("Right axis value"=w336, "Left axis value"=w335, "RobotDriveDevRef"=w345) -> ()  [unwired: 6 in, 3 out]
            n221 = call "Elapsed Time"() -> ("Time has Elapsed"=w334:bool)  [unwired: 12 in, 7 out]
            n222 = Wait (ms)(milliseconds to wait=u32 50) -> ()  [unwired: 1 out]
          }
        }
        frame #4 {
          n223 = while {
            stop <- w357 stop-if-true
            n224 = local read "Aiming Gains"() -> (w347:T1)
            n225 = global read "Robot Global Data.vi" "T1 X"() -> (w355:dbl)
            n226 = Absolute Value(x=w355) -> (abs(x)=w360:dbl)
            n227 = Less?(x=w360, y=0.05) -> (x < y?=w358:bool)
            n228 = call-poly <vilib>:"PID.vi"("output range"=cluster{"output high":dbl, "output low":dbl} {"output high"=0.7, "output low"=-0.7}, "PID gains"=w347, "process variable"=w355, "setpoint"=0.0) -> ("output"=w349:dbl)  [unwired: 6 in, 1 out]
            n229 = case shown="False" w358 {
              tunnel: [FALSE FALSE] -> w357
              frame False {
              }
              frame True {
              }
            }
            n230 = Multiply(x=w349, y=-1.0) -> (x*y=w348:dbl)
            n231 = call <vilib>:"WPI_RobotDriveRefNum Registry Get.vi"("refnum name"="Left and Right Motors") -> ("RobotDriveDevRef"=w351:T11)  [unwired: 9 in, 1 out]
            n232 = call <vilib>:"WPI_RobotDriveTankDrive.vi"("Right axis value"=w348, "Left axis value"=w349, "RobotDriveDevRef"=w351) -> ()  [unwired: 6 in, 3 out]
            n233 = Wait (ms)(milliseconds to wait=u32 50) -> ()  [unwired: 1 out]
          }
        }
      }
    }
    frame "Dashboard Auton" {
      n234 = flat-sequence {
        frame #0 {
          n235 = while {
            stop <- w373 stop-if-true
            n236 = global read "Robot Global Data.vi" "T1 X"() -> (w371:dbl)
            n237 = Absolute Value(x=w371) -> (abs(x)=w376:dbl)
            n238 = Less?(x=w376, y=0.05) -> (x < y?=w374:bool)
            n239 = call-poly <vilib>:"PID.vi"("output range"=cluster{"output high":dbl, "output low":dbl} {"output high"=0.7, "output low"=-0.7}, "PID gains"="Aiming Gains", "process variable"=w371, "setpoint"=0.0) -> ("output"=w364:dbl)  [unwired: 6 in, 1 out]
            n240 = case shown="False" w374 {
              tunnel: [FALSE FALSE] -> w373
              frame False {
              }
              frame True {
              }
            }
            n241 = Multiply(x=w364, y=-1.0) -> (x*y=w363:dbl)
            n242 = call <vilib>:"WPI_RobotDriveRefNum Registry Get.vi"("refnum name"="Left and Right Motors") -> ("RobotDriveDevRef"=w366:T11)  [unwired: 9 in, 1 out]
            n243 = call <vilib>:"WPI_RobotDriveTankDrive.vi"("Right axis value"=w363, "Left axis value"=w364, "RobotDriveDevRef"=w366) -> ()  [unwired: 6 in, 3 out]
            n244 = Wait (ms)(milliseconds to wait=u32 50) -> ()  [unwired: 1 out]
          }
        }
      }
    }
  }
